vi "batchQueuesCommands.vi"(8 "error in (no error)":errorcluster, 9 "Batch parameters":T1, 11 "QueueMessages":refnum<queue>) -> (0 "error out":errorcluster)   [LabVIEW 2023]
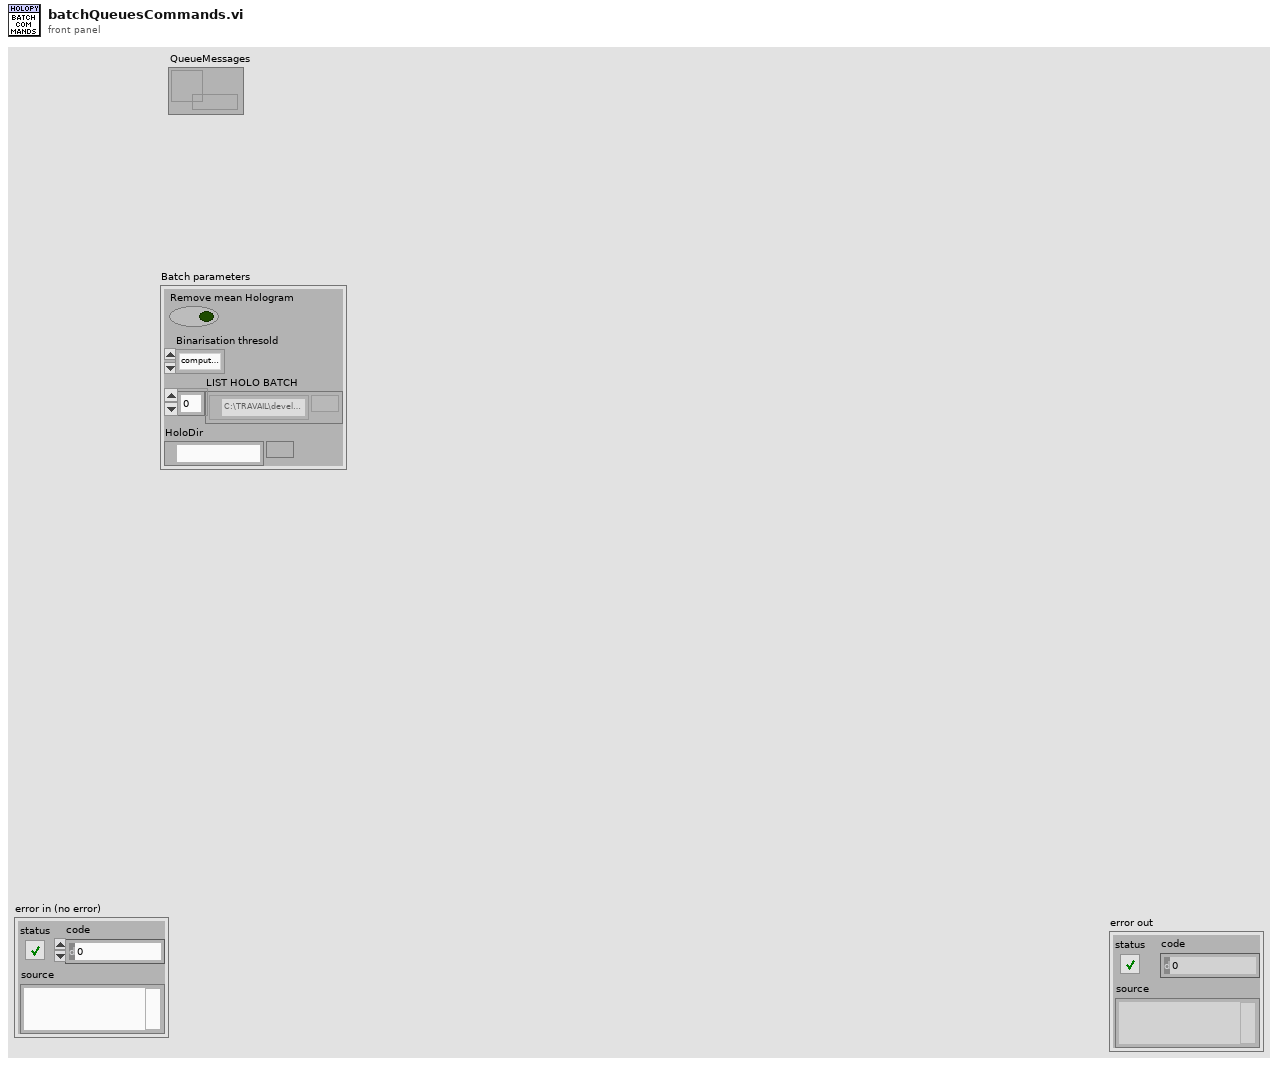
[diagram p1: front panel]
types:
  T1 = cluster{"Remove mean Hologram":bool, "Binarisation thresold ":enum16{"compute on 1st hologram", "compute on each hologram"}, "LIST HOLO BATCH":path[], "HoloDir":path}
  T2 = enum16{"compute on 1st hologram", "compute on each hologram"}
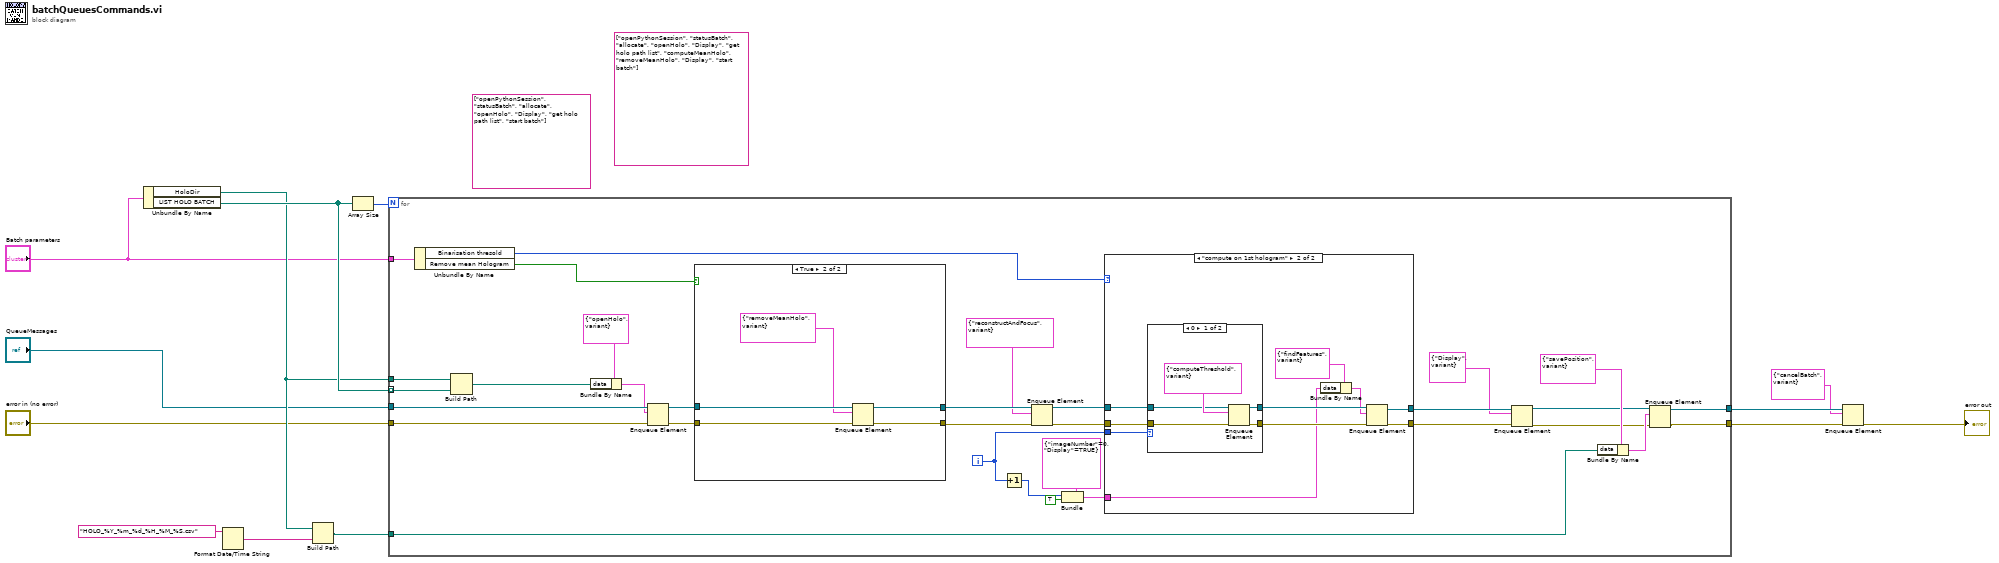
[diagram p0: block diagram]
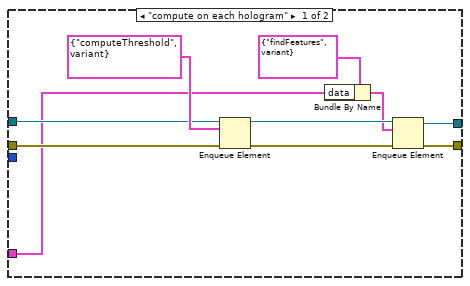
[diagram p2: hidden frame]
diagram:
  (unwired) string[] ["openPythonSession", "statusBatch", "allocate", "openHolo", "Display", "get holo path list", "start batch"]
  (unwired) string[] ["openPythonSession", "statusBatch", "allocate", "openHolo", "Display", "get holo path list", "computeMeanHolo", "removeMeanHolo", "Display", "start batch"]
  n1 = Unbundle By Name("Batch parameters") -> ("HoloDir"=w8:path, "LIST HOLO BATCH"=w10:path[])
  n2 = Format Date/Time String(time format string (%c)="HOLO_%Y_%m_%d_%H_%M_%S.csv") -> (date/time string=w12:string)  [unwired: 2 in]
  n3 = Build Path(base path=w8, name or relative path=w12) -> (appended path=w9:path)
  n4 = Array Size(array=w10) -> (size(s)=w11:i32)
  n5 = for {
    N: w11 -> [_]
    tunnel: w10 -> [w26] mode=indexing
    tunnel: "QueueMessages" -> [w45]
    tunnel: "error in (no error)" -> [w44]
    tunnel: "Batch parameters" -> [w41]
    tunnel: [w31] -> w6
    tunnel: [w30] -> w7
    tunnel: w9 -> [w27]
    tunnel: w8 -> [w25]
    i -> [w21]
    n6 = Unbundle By Name(w41) -> ("Binarisation thresold"=w34:T2, "Remove mean Hologram"=w38:bool)
    n7 = Build Path(base path=w25, name or relative path=w26) -> (appended path=w19:path)
    n8 = Bundle By Name(cluster=cluster{"command":string, "data":variant} {"command"="openHolo", "data"=variant} ("element"), "data"=w19) -> (w42:cluster{"command":string, "data":variant})
    n9 = Enqueue Element(queue=w45, element=w42, error in (no error)=w44) -> (queue out=w39:refnum<queue>, error out=w40:errorcluster)  [unwired: 1 in, 1 out]
    n10 = case shown="True" w38 {
      tunnel: w40 -> [w73 w79]
      tunnel: w39 -> [w74 w78]
      tunnel: [w74 w77] -> w37
      tunnel: [w73 w76] -> w36
      frame False {
      }
      frame True {
        n11 = Enqueue Element(queue=w78, element=cluster{"command":string, "data":variant} {"command"="removeMeanHolo", "data"=variant}, error in (no error)=w79) -> (queue out=w77:refnum<queue>, error out=w76:errorcluster)  [unwired: 1 in, 1 out]
      }
    }
    n12 = Increment(x=w21) -> (x+1=w22:i32)
    n13 = Enqueue Element(queue=w37, element=cluster{"command":string, "data":variant} {"command"="reconstructAndFocus", "data"=variant}, error in (no error)=w36) -> (queue out=w32:refnum<queue>, error out=w33:errorcluster)  [unwired: 1 in, 1 out]
    n14 = Bundle(cluster=cluster{"imageNumber":u32, "Display":bool} {"imageNumber"=0, "Display"=TRUE}, "imageNumber"=w22, "Display"=TRUE) -> (w24:cluster{"imageNumber":u32, "Display":bool})
    n15 = case shown="\"compute on 1st hologram\"" w34 {
      tunnel: w33 -> [w50 w61]
      tunnel: w32 -> [w49 w60]
      tunnel: [w47 w59] -> w17
      tunnel: [w48 w58] -> w18
      tunnel: w24 -> [w46 w57]
      tunnel: w21 -> [_ w56]
      frame "compute on each hologram" {
        n16 = Enqueue Element(queue=w49, element=cluster{"command":string, "data":variant} {"command"="computeThreshold", "data"=variant}, error in (no error)=w50) -> (queue out=w54:refnum<queue>, error out=w55:errorcluster)  [unwired: 1 in, 1 out]
        n17 = Bundle By Name(cluster=cluster{"command":string, "data":variant} {"command"="findFeatures", "data"=variant} ("element"), "data"=w46) -> (w53:cluster{"command":string, "data":variant})
        n18 = Enqueue Element(queue=w54, element=w53, error in (no error)=w55) -> (queue out=w47:refnum<queue>, error out=w48:errorcluster)  [unwired: 1 in, 1 out]
      }
      frame "compute on 1st hologram" {
        n19 = case shown="0" w56 {
          tunnel: [w70 w71] -> w65
          tunnel: [w69 w72] -> w64
          tunnel: w61 -> [w67 w71]
          tunnel: w60 -> [w66 w72]
          frame 0 {
            n20 = Enqueue Element(queue=w66, element=cluster{"command":string, "data":variant} {"command"="computeThreshold", "data"=variant}, error in (no error)=w67) -> (queue out=w69:refnum<queue>, error out=w70:errorcluster)  [unwired: 1 in, 1 out]
          }
          frame 1, Default {
          }
        }
        n21 = Bundle By Name(cluster=cluster{"command":string, "data":variant} {"command"="findFeatures", "data"=variant} ("element"), "data"=w57) -> (w63:cluster{"command":string, "data":variant})
        n22 = Enqueue Element(queue=w64, element=w63, error in (no error)=w65) -> (queue out=w59:refnum<queue>, error out=w58:errorcluster)  [unwired: 1 in, 1 out]
      }
    }
    n23 = Enqueue Element(queue=w17, element=cluster{"command":string, "data":variant} {"command"="Display", "data"=variant}, error in (no error)=w18) -> (queue out=w16:refnum<queue>, error out=w15:errorcluster)  [unwired: 1 in, 1 out]
    n24 = Bundle By Name(cluster=cluster{"command":string, "data":variant} {"command"="savePosition", "data"=variant} ("element"), "data"=w27) -> (w28:cluster{"command":string, "data":variant})
    n25 = Enqueue Element(queue=w16, element=w28, error in (no error)=w15) -> (queue out=w31:refnum<queue>, error out=w30:errorcluster)  [unwired: 1 in, 1 out]
  }
  n26 = Enqueue Element(queue=w6, element=cluster{"command":string, "data":variant} {"command"="cancelBatch", "data"=variant}, error in (no error)=w7) -> (error out=→"error out":errorcluster)  [unwired: 1 in, 2 out]
